vi "Open.vi"   [LabVIEW 2017, in "VILauncher.lvlib"]
doc: "This VI is polymorphic, it opens a reference to a dynamic VI either specified by path (<B>VI path</B>) or by reference (<B>VI refnum</B>) and returns the reference to the opened VI in <B>VI refnum out</B>. Remember to close the VI reference when you're done using it.\n\nThe optional <B>Application reference</B> can be used to specify another application instance to open the VI reference in. Use the Open Application Reference LabVIEW function to open another application reference.\n\nUse the optional <B>Reentrancy mode</B> input to specify whether the dynamic VI should be opened as a reentrant or a non-reentrant instance. Set this to Auto (default) to first try as reentrant, and if that fails, as non-reentrant. The <B>VI refnum opened as reentrant?</B> output will reflect the instantiation mode.\n\nThe <B>VI refnum opened?</B> output will only be True if the dynamic VI's <B>Last execution state</B> is \"Idle\" or \"Running\".\n\nThis VI is reentrant, and it doesn't run if there is an error on <B>Error in</B>.\n\nSteen Schmidt\nGPower"
uses:
  VILauncher.lvlib
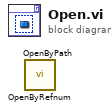
[diagram p0: block diagram]
diagram:
  n1 = call "OpenByRefnum.vi"() -> ()  [unwired: 11 in, 5 out]
  n2 = call "OpenByPath.vi"() -> ()  [unwired: 11 in, 5 out]
